vi "VG_ISOmin_P.vi"() -> ()   [LabVIEW 2020]
panel:
  out "ISOM CF":dbl
  out "ISOP CF":dbl
  out "ISOM CO":dbl
  out "ISOP CO":dbl
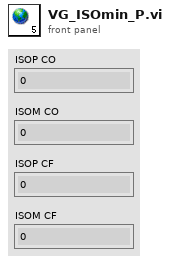
[diagram p1: front panel]
diagram:
